vi "Get Pane Control Refnums by Names.vi"(8 "error in":errorcluster, 9 "Selection":T1(ring), 10 "Control Labels":string[](array[string]), 11 "Pane Refnum":refnum<vi>) -> (0 "error out":errorcluster, 1 "All Ctls found?":bool, 2 "Ctl Refnums":refnum<vi>[](array[refnum]))   [LabVIEW 2021, in "Utilities.lvlib"]
doc: "Returns an array of control refnums, labels and data, from the front panel of the calling VI.\n\nThis VI also accounts for tab controls within other tab controls."
uses:
  Utilities.lvlib
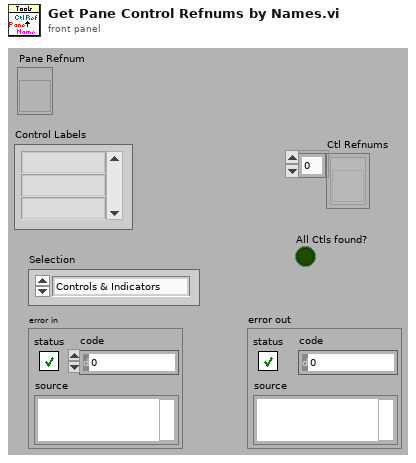
[diagram p1: front panel]
types:
  T1 = enum16{"Controls & Indicators", "Controls", "Indicators"}
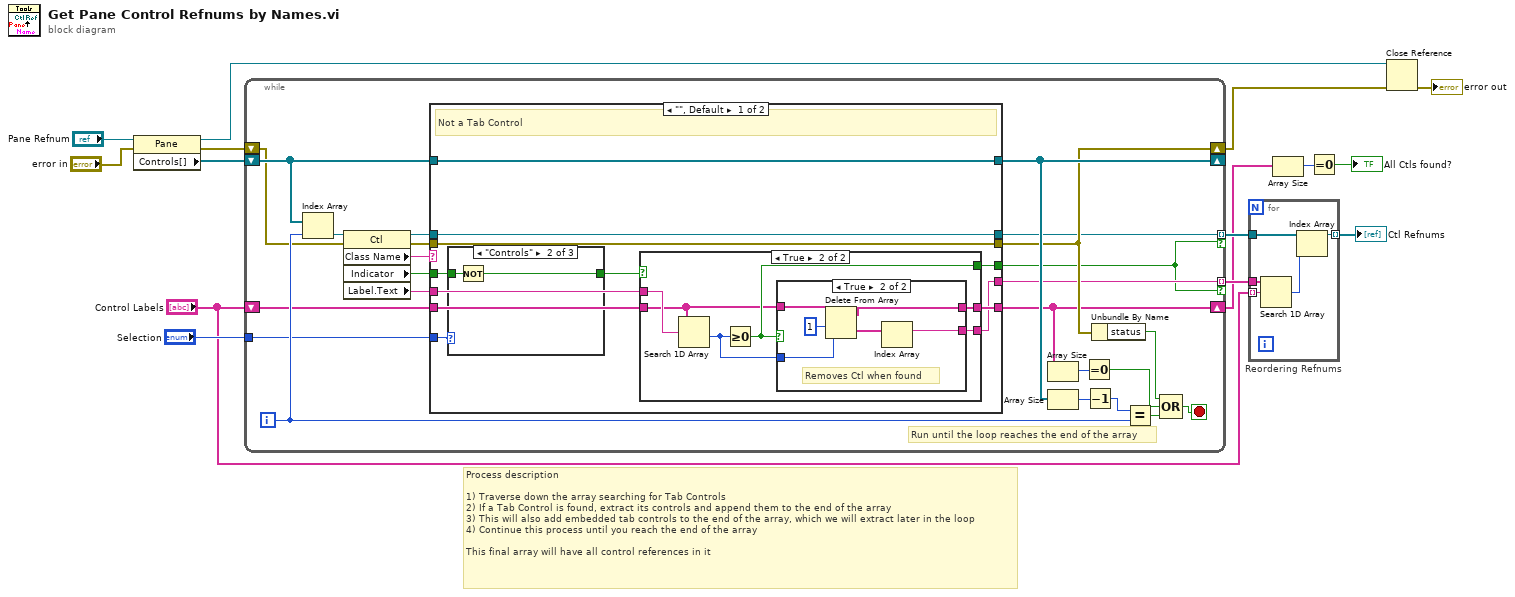
[diagram p0: block diagram]
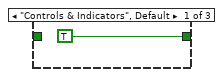
[diagram p4: hidden frame]
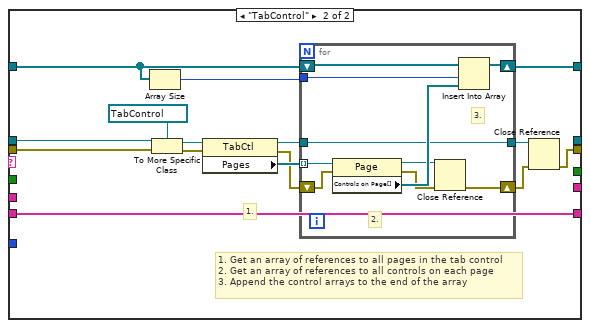
[diagram p6: hidden frame]
diagram:
  # "Process description\n\n1) Traverse down the array searching for Tab Controls\n2) If a Tab Control is found, extract its controls and append them to the end of the array\n3) This will also add embedded tab controls to the end of the array, which we will extract later in the loop\n4) Continue this process until you reach the end of the array\n\nThis final array will have all control references in it"
  n1 = property class="Pane"(reference="Pane Refnum", error in="error in") -> (reference out=w14:refnum<vi>, error out=w15:errorcluster, "Controls[]"=w2:refnum<vi>[])
  n2 = while {
    shift-right: [w32] -> _
    shift-left: w2 -> [w38]
    shift-right: [w29] -> w13
    shift-left: w15 -> [w31]
    shift-right: [w22] -> w4
    shift-left: "Control Labels" -> [w24]
    tunnel: [w23] -> w8 mode=indexing if=w16
    tunnel: "Selection" -> [w18]
    tunnel: [w17] -> w5 mode=indexing if=w16
    i -> [w33]
    stop <- w27 stop-if-true
    # "Run until the loop reaches the end of the array"
    n3 = Index Array(array=w38, index=w33) -> (element=w34:refnum<vi>)
    n4 = property class="Ctl"(reference=w34, error in=w31) -> (reference out=w39:refnum<vi>, error out=w30:errorcluster, "Class Name"=w37:string, "Indicator"=w19:bool, "Label.Text"=w25:string)
    n5 = case shown="\"\", Default" w37 {
      tunnel: w39 -> [w47 w83]
      tunnel: w38 -> [w50 w79]
      tunnel: [w50 w80] -> w32
      tunnel: w30 -> [w49 w76]
      tunnel: [w49 w72] -> w29
      tunnel: w25 -> [w48 _]
      tunnel: w24 -> [w45 w69]
      tunnel: [w47 _] -> w23
      tunnel: [w46 _] -> w16
      tunnel: [w44 w69] -> w22
      tunnel: w19 -> [w42 _]
      tunnel: w18 -> [w43 _]
      tunnel: [w40 _] -> w17
      frame "", Default {
        # "Not a Tab Control"
        n6 = case shown="\"Controls\"" w43 {
          tunnel: w42 -> [_ w67 w68]
          tunnel: [TRUE ("Indicator") w66 w68] -> w41
          frame "Controls & Indicators", Default {
          }
          frame "Controls" {
            n7 = Not(x=w67) -> (.not. x?=w66:bool)
          }
          frame "Indicators" {
          }
        }
        n8 = case shown="True" w41 {
          tunnel: w48 -> [_ w57]
          tunnel: [_ w56] -> w46
          tunnel: w45 -> [w51 w55]
          tunnel: [w51 w53] -> w44
          tunnel: [_ w52] -> w40
          frame False {
          }
          frame True {
            n9 = Search 1D Array(1D array=w55, element=w57) -> (index of element=w54:i32)  [unwired: 1 in]
            n10 = Greater Or Equal To 0?(x=w54) -> (x >= 0?=w56:bool)
            n11 = case shown="True" w56 {
              tunnel: w55 -> [w58 w64]
              tunnel: w54 -> [_ w63]
              tunnel: [w58 w61] -> w53
              tunnel: [_ w59] -> w52
              frame False {
              }
              frame True {
                # "Removes Ctl when found"
                n12 = Delete From Array(array=w64, length=1, index=w63) -> (deleted portion=w60:string[], array with subset deleted=w61:string[])
                n13 = Index Array(array=w60) -> (element=w59:string)  [unwired: 1 in]
              }
            }
          }
        }
      }
      frame "TabControl" {
        # "1. Get an array of references to all pages in the tab control\n2. Get an array of references to all controls on each page\n3. Append the control arrays to the end of the array"
        # "1."
        n14 = Array Size(array=w79) -> (size(s)=w77:i32)
        n15 = To More Specific Class(target class=refnum<vi> refnum ("Tab Control"), reference=w83, error in=w76) -> (specific class reference=w82:refnum<vi>, error out=w75:errorcluster)
        n16 = property class="TabCtl"(reference=w82, error in=w75) -> (reference out=w73:refnum<vi>, error out=w74:errorcluster, "Pages"=w81:refnum<vi>[])
        n17 = for {
          tunnel: w81 -> [w93] mode=indexing
          tunnel: w77 -> [w91]
          shift-right: [w92] -> w80
          shift-left: w79 -> [w90]
          tunnel: w73 -> [w87]
          tunnel: [w87] -> w71
          shift-right: [w84] -> w70
          shift-left: w74 -> [w88]
          # "3."
          # "2."
          n18 = property class="Page"(reference=w93, error in=w88) -> (reference out=w86:refnum<vi>, error out=w85:errorcluster, "Controls on Page[]"=w89:refnum<vi>[])
          n19 = Close Reference(reference=w86, error in (no error)=w85) -> (error out=w84:errorcluster)
          n20 = Insert Into Array(array=w90, index=w91, new element=w89) -> (w92:refnum<vi>[])
        }
        n21 = Close Reference(reference=w71, error in (no error)=w70) -> (error out=w72:errorcluster)
      }
    }
    n22 = Array Size(array=w22) -> (size(s)=w21:i32)
    n23 = Array Size(array=w32) -> (size(s)=w36:i32)
    n24 = Equal To 0?(x=w21) -> (x = 0?=w20:bool)
    n25 = Decrement(x=w36) -> (x-1=w35:i32)
    n26 = Unbundle By Name(w29) -> ("status"=w26:bool)
    n27 = Equal?(x=w35, y=w33) -> (x = y?=w28:bool)
    n28 = Compound Arithmetic op=OR(w26, w20, w28) -> (w27:bool)
  }
  n29 = for "Reordering Refnums" {
    tunnel: w8 -> [w98]
    tunnel: [w96] -> w7 mode=indexing
    tunnel: "Control Labels" -> [w95] mode=indexing
    tunnel: w5 -> [w94]
    n30 = Search 1D Array(1D array=w94, element=w95) -> (index of element=w97:i32)  [unwired: 1 in]
    n31 = Index Array(array=w98, index=w97) -> (element=w96:refnum<vi>)
  }
  "Ctl Refnums" <- w7
  n32 = Array Size(array=w4) -> (size(s)=w11:i32)
  n33 = Equal To 0?(x=w11) -> (x = 0?=→"All Ctls found?":bool)
  n34 = Close Reference(reference=w14, error in (no error)=w13) -> (error out=→"error out":errorcluster)
